vi "run.create_commit.vi"(8 "error in":errorcluster, 11 "RunCreateStaging in":refnum<class "RunCreateStaging.lvclass">) -> (0 "error out":errorcluster, 2 "Run":refnum<class "Run.lvclass">, 3 "RunCreateStaging out":refnum<class "RunCreateStaging.lvclass">)   [LabVIEW 2020, in "RunCreateStaging.lvclass"]
doc: "Creates the staged run in Nominal and returns a handle to it."
uses:
  RunCreateStaging.lvclass
  Run/Run.lvclass
  RunCreateStaging.lvclass/RunCreateStaging.ctl
  Client/Client.lvclass/Client.ctl
  Run/Run.lvclass/Run.ctl
  client.lvlib
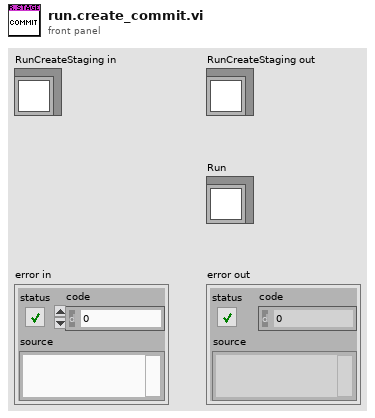
[diagram p1: front panel]
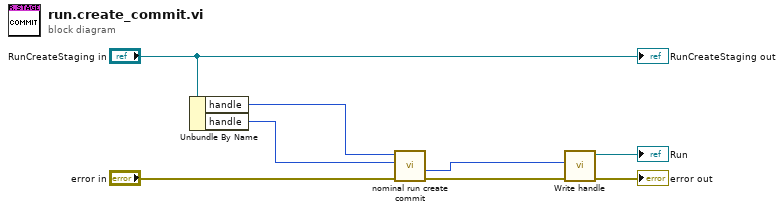
[diagram p0: block diagram]
diagram:
  n1 = Unbundle By Name("RunCreateStaging in") -> ("handle"=w1:i32, "handle"=w6:i32)
  n2 = call "nominal run create commit.vi"("error in (no error)"="error in", "staging"=w6, "client"=w1) -> ("error out"=w3:errorcluster, "out_run out"=w5:i32)  [unwired: 6 in, 1 out]
  n3 = call "Write handle.vi"("error in (no error)"=w3, "handle"=w5) -> ("error out"=→"error out":errorcluster, "Run out"=→"Run":refnum<class "Run.lvclass">)  [unwired: 8 in]
  "RunCreateStaging out" <- "RunCreateStaging in"
